vi "case1_selector.vi"(0 "T1":dbl, 2 "T2":dbl, 3 "Delay":dbl) -> (6 "Case 1 selector":enum16{"D<=T1-T2", "T1-T2<D<T1", "D>=T1"}(ring))   [LabVIEW 2015]
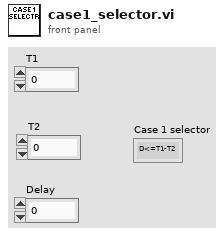
[diagram p1: front panel]
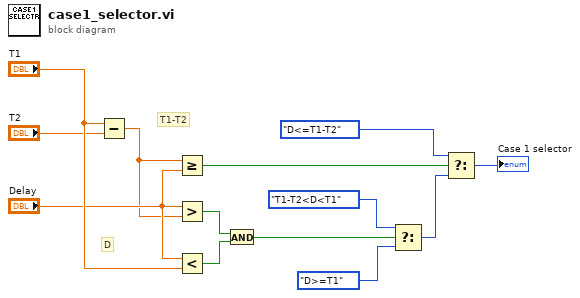
[diagram p0: block diagram]
diagram:
  # "T1-T2"
  # "D"
  n1 = Subtract(x="T1", y="T2") -> (x-y=w5:dbl)
  n2 = Greater Or Equal?(x=w5, y="Delay") -> (x >= y?=w3:bool)
  n3 = Greater?(x="Delay", y=w5) -> (0:w6:bool)
  n4 = Less?(x="Delay", y="T1") -> (x < y?=w9:bool)
  n5 = And(x=w6, y=w9) -> (x .and. y?=w10:bool)
  n6 = Select(t=enum16{"D<=T1-T2", "T1-T2<D<T1", "D>=T1"}."T1-T2<D<T1", s=w10, f=enum16{"D<=T1-T2", "T1-T2<D<T1", "D>=T1"}."D>=T1") -> (s? t:f=w13:enum16{"D<=T1-T2", "T1-T2<D<T1", "D>=T1"})
  n7 = Select(t=enum16{"D<=T1-T2", "T1-T2<D<T1", "D>=T1"}."D<=T1-T2", s=w3, f=w13) -> (s? t:f=→"Case 1 selector":enum16{"D<=T1-T2", "T1-T2<D<T1", "D>=T1"})
